vi "VerifyLicense.vi"(6 "Tips":bool caption="启用", 9 "UID":string, 10 "License":string) -> (1 "LicenOut":string, 2 "user":string)   [LabVIEW 2015]
panel:
  in  "用户级别":u16(ring) items=["普通用户", "VIP", "SVIP"]
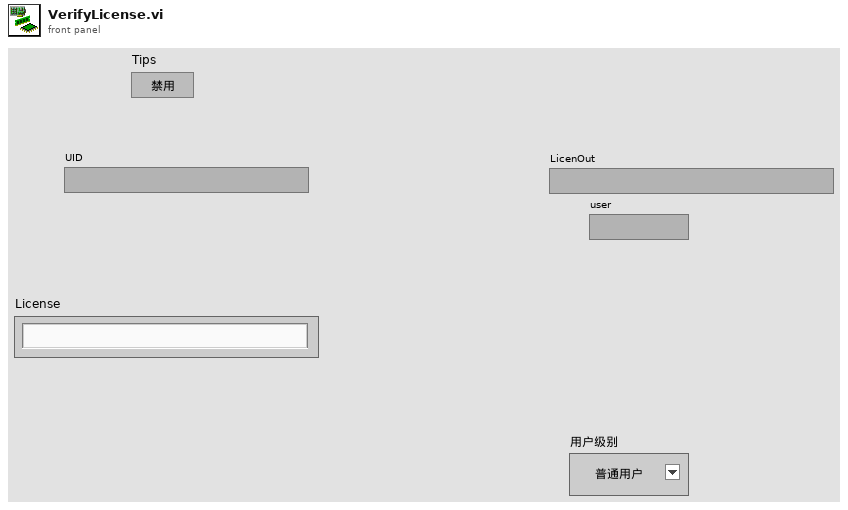
[diagram p1: front panel]
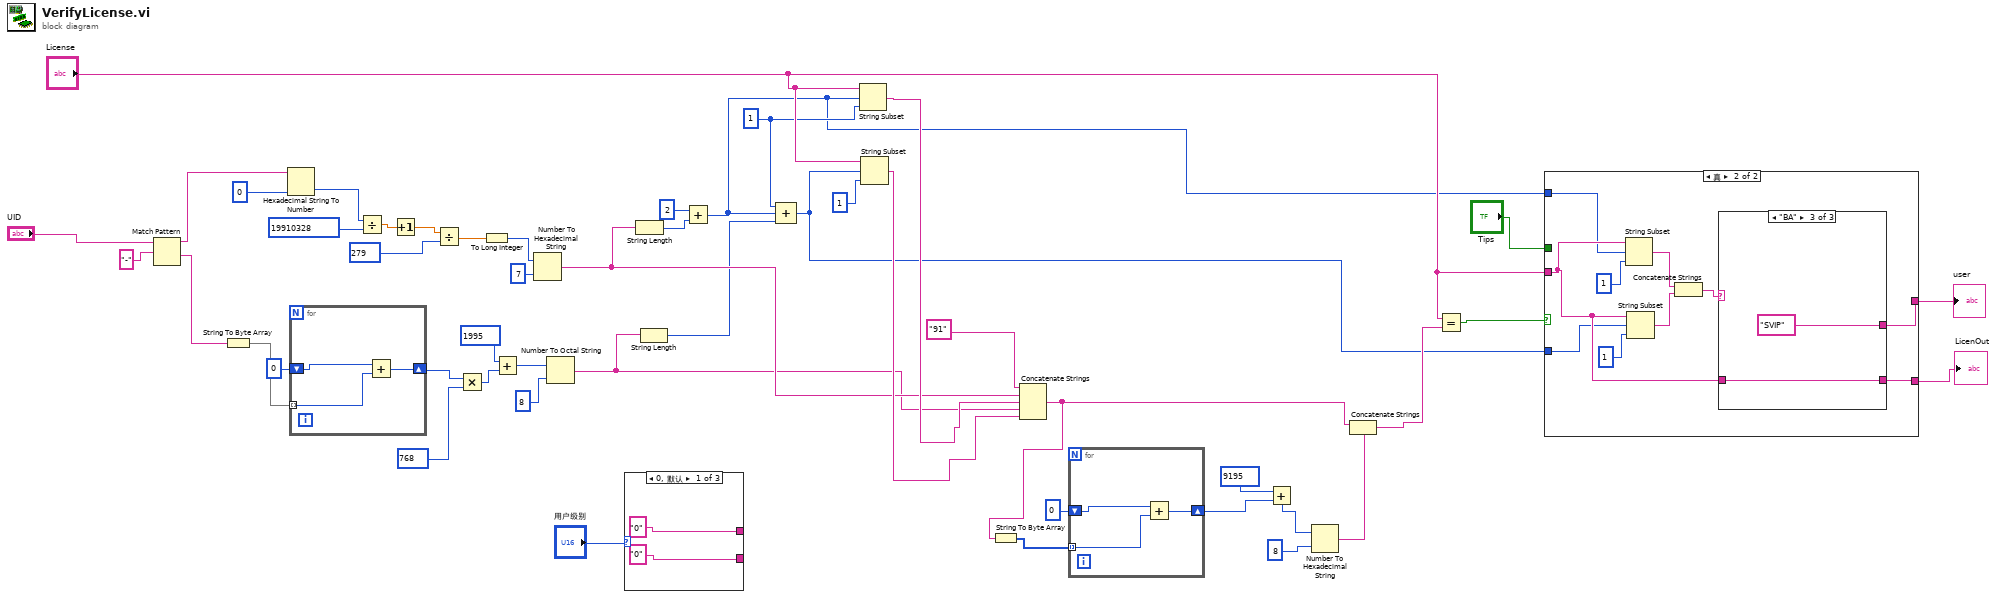
[diagram p0: block diagram]
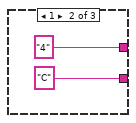
[diagram p2: hidden frame]
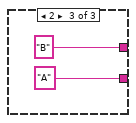
[diagram p3: hidden frame]
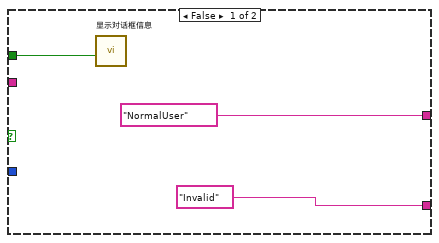
[diagram p4: hidden frame]
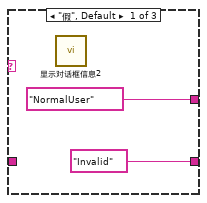
[diagram p5: hidden frame]
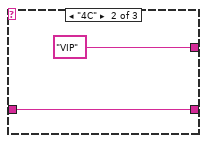
[diagram p6: hidden frame]
diagram:
  w4 = 1 ("长度（剩余）")
  n1 = Match Pattern(string="UID", regular expression="-" ("字符串")) -> (before substring=w26:string, after substring=w25:string)  [unwired: 1 in, 2 out]
  n2 = String To Byte Array(string=w25) -> (unsigned byte array=w40:u8[])
  n3 = Hexadecimal String To Number(string=w26, default (0uL)=u64 0 ("默认(0 U32)")) -> (number=w47:u64)  [unwired: 1 in, 1 out]
  n4 = for {
    tunnel: w40 -> [w51] mode=indexing
    shift-right: [w50] -> w38
    shift-left: u8 0 -> [w49]
    n5 = Add(x=w49, y=w51) -> (x+y=w50:u8)
  }
  n6 = Divide(x=w47, y=19910328) -> (x/y=w45:dbl)
  n7 = Increment(x=w45) -> (x+1=w44:dbl)
  n8 = Divide(x=w44, y=279) -> (x/y=w42:dbl)
  n9 = Multiply(x=w38, y=768) -> (x*y=w34:i32)
  n10 = To Long Integer(number=w42) -> (32bit integer=w41:i32)
  n11 = Add(x=1995, y=w34) -> (x+y=w35:i32)
  n12 = Number To Hexadecimal String(1:i16 7 ("宽度(-)"), 2:w41) -> (0:w8:string)
  n13 = Number To Octal String(1:i16 8 ("宽度(-)"), 2:w35) -> (0:w5:string)
  n14 = case shown="0, 默认" "用户级别" {
    tunnel: ["0" "4" "B"] -> _
    tunnel: ["0" "C" "A"] -> _
    frame 0, Default {
    }
    frame 1 {
    }
    frame 2 {
    }
  }
  n15 = String Length(string=w8) -> (length=w7:i32)
  n16 = String Length(string=w5) -> (length=w3:i32)
  n17 = Add(x=2, y=w7) -> (x+y=w2:i32)
  n18 = Compound Arithmetic op=ADD(w4, w2, w3) -> (w1:i32)
  n19 = String Subset(string="License", offset (0)=w2, length (rest)=w4) -> (substring=w12:string)
  n20 = String Subset(string="License", offset (0)=w1, length (rest)=1 ("长度（剩余）")) -> (substring=w11:string)
  n21 = Concatenate Strings("91", w8, w12, w5, w11) -> (w16:string)
  n22 = String To Byte Array(string=w16) -> (unsigned byte array=w29:u8[])
  n23 = for {
    tunnel: w29 -> [w60] mode=indexing
    shift-right: [w59] -> w19
    shift-left: 0 -> [w58]
    n24 = Add(x=w58, y=w60) -> (x+y=w59:i32)
  }
  n25 = Add(x=9195, y=w19) -> (x+y=w18:i32)
  n26 = Number To Hexadecimal String(1:i16 8 ("宽度(-)"), 2:w18) -> (0:w23:string)
  n27 = Concatenate Strings(w16, w23) -> (w22:string)
  n28 = Equal?(x="License", y=w22) -> (x = y?=w21:bool)
  n29 = case shown="真" w21 {
    tunnel: ["NormalUser" w73] -> w20
    tunnel: "License" -> [_ w66]
    tunnel: ["Invalid" w67] -> w10
    tunnel: "Tips" -> [w61 _]
    tunnel: w2 -> [_ w65]
    tunnel: w1 -> [_ w64]
    frame False {
      n30 = call "显示对话框信息"("Enable"=w61) -> ()  [unwired: 9 in, 2 out]
    }
    frame True {
      n31 = String Subset(string=w66, offset (0)=w65, length (rest)=1 ("长度（剩余）")) -> (substring=w71:string)
      n32 = String Subset(string=w66, offset (0)=w64, length (rest)=1 ("长度（剩余）")) -> (substring=w69:string)
      n33 = Concatenate Strings(w71, w69) -> (w68:string)
      n34 = case shown="\"BA\"" w68 {
        tunnel: ["NormalUser" "VIP" "SVIP"] -> w73
        tunnel: ["Invalid" w76 w78] -> w67
        tunnel: w66 -> [_ w76 w78]
        frame "假", Default {
          n35 = call "显示对话框信息2"() -> ()  [unwired: 10 in, 2 out]
        }
        frame "4C" {
        }
        frame "BA" {
        }
      }
    }
  }
  "LicenOut" <- w10
  "user" <- w20
